vi "KH TURCK ETHERNETIP IOL WordToByte.vi"(11 "TBEN-S2-4IOL Output Values Word":u16[](array[numeric])) -> (3 "TBEN-S2-4IOL Output Values Bytes":u8[](array[numeric]))   [LabVIEW 2021]
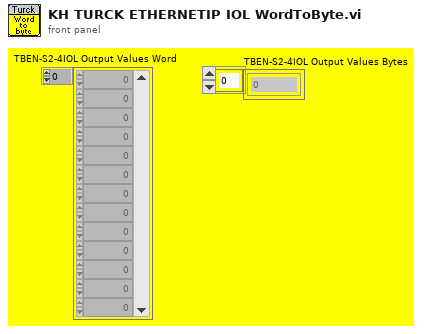
[diagram p1: front panel]
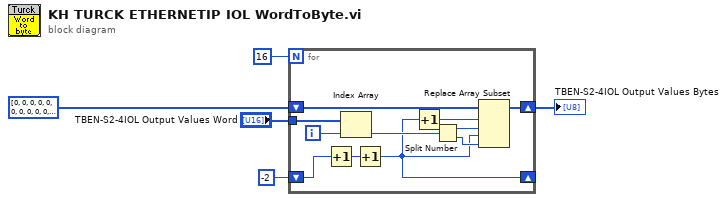
[diagram p0: block diagram]
diagram:
  n1 = for {
    N: 16 -> [_]
    shift-right: [w15] -> w2
    shift-left: u8[] [0, 0, 0, 0, 0, 0, 0, 0, 0, 0, 0, 0, 0, 0, 0, 0] ("Data") -> [w16]
    tunnel: "TBEN-S2-4IOL Output Values Word" -> [w11]
    shift-right: [w8] -> _
    shift-left: -2 ("Numeric") -> [w7]
    i -> [w9]
    n2 = Increment(x=w7) -> (x+1=w6:i32)
    n3 = Index Array(array=w11, index=w9) -> (element=w12:u16)
    n4 = Increment(x=w6) -> (x+1=w8:i32)
    n5 = Increment(x=w8) -> (x+1=w10:i32)
    n6 = Split Number(x=w12) -> (hi(x)=w14:u8, lo(x)=w13:u8)
    n7 = Replace Array Subset(array=w16, new element #1=w14, index #1=w10, new element #2=w13, index #2=w8) -> (w15:u8[])
  }
  "TBEN-S2-4IOL Output Values Bytes" <- w2
